vi "Check if Cluster Control.vi"(0 "Typedef Cluster":refnum<vi>, 1 "String Controls in":string[](array[string]), 2 "Controls Ref IN":refnum<vi>[](array[refnum]), 7 "Ctl Refnum":refnum<vi>, 9 "vi reference":refnum<vi>, 11 "error in":errorcluster) -> (4 "Controls Ref Out":refnum<vi>[](array[refnum]), 6 "String Controls out":string[](array[string]), 15 "error out":errorcluster)   [LabVIEW 2021, in "Converter.lvlib"]
uses:
  Converter.lvlib
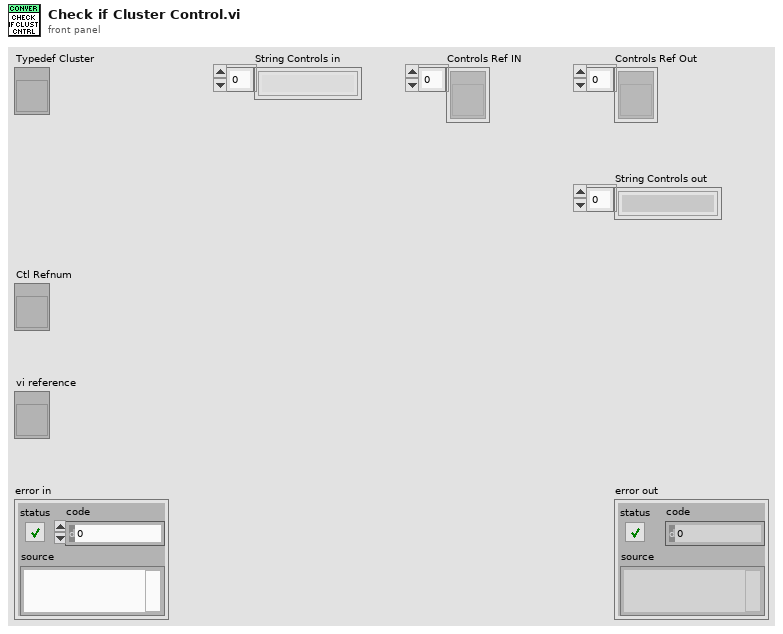
[diagram p1: front panel]
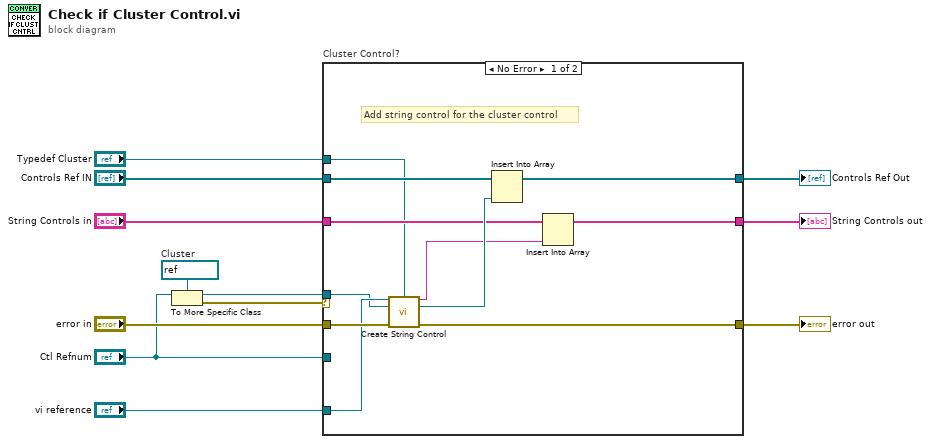
[diagram p0: block diagram]
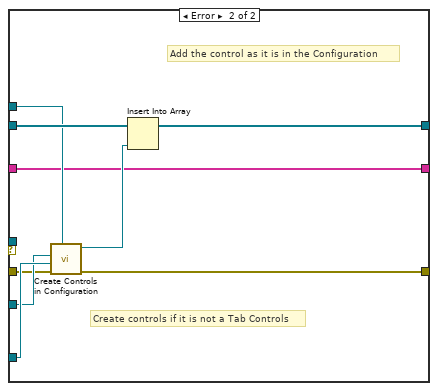
[diagram p2: hidden frame]
diagram:
  w8 = refnum<vi> refnum  # Cluster
  n1 = To More Specific Class(target class=w8, reference="Ctl Refnum") -> (specific class reference=w10:refnum<vi>, error out=w9:errorcluster)  [unwired: 1 in]
  n2 = case "Cluster Control?" shown="No Error" w9 {
    tunnel: "Controls Ref IN" -> [w19 w32]
    tunnel: [w18 w31] -> w3
    tunnel: "vi reference" -> [w21 w30]
    tunnel: [w22 w28] -> w5
    tunnel: "Typedef Cluster" -> [w13 w27]
    tunnel: "Ctl Refnum" -> [_ w26]
    tunnel: "error in" -> [w23 w25]
    tunnel: w10 -> [w20 _]
    tunnel: [w15 w24] -> w11
    tunnel: "String Controls in" -> [w16 w24]
    frame No Error {
      # "Add string control for the cluster control"
      n3 = call "Create String Control.vi"("VI Refnum"=w21, "Typedef Cluster"=w13, "Clust Refnum"=w20, "error in (no error)"=w23) -> ("Reference String"=w14:string, "String ctl ref"=w17:refnum<vi>, "error out"=w22:errorcluster)  [unwired: 9 in]
      n4 = Insert Into Array(array=w19, new element=w17) -> (w18:refnum<vi>[])  [unwired: 1 in]
      n5 = Insert Into Array(array=w16, new element=w14) -> (w15:string[])  [unwired: 1 in]
    }
    frame Error {
      # "Add the control as it is in the Configuration"
      # "Create controls if it is not a Tab Controls"
      n6 = call "Create Controls in Configuration.vi"("error in (no error)"=w25, "VI Refnum"=w30, "Ctl Refnum"=w26, "Cluster Ref"=w27) -> ("error out"=w28:errorcluster, "Control out"=w29:refnum<vi>)  [unwired: 6 in]
      n7 = Insert Into Array(array=w32, new element=w29) -> (w31:refnum<vi>[])  [unwired: 1 in]
    }
  }
  "String Controls out" <- w11
  "error out" <- w5
  "Controls Ref Out" <- w3
